vi "add_PointCloud_roslv.vi"(3 "channels":cluster{"name":string, "values":sgl[]}[](array[cluster]), 4 "points":cluster{"x":sgl, "y":sgl, "z":sgl}[](array[cluster]), 5 "frame_id":string, 6 "msg in":string) -> (2 "msg out":string)   [LabVIEW 2014]
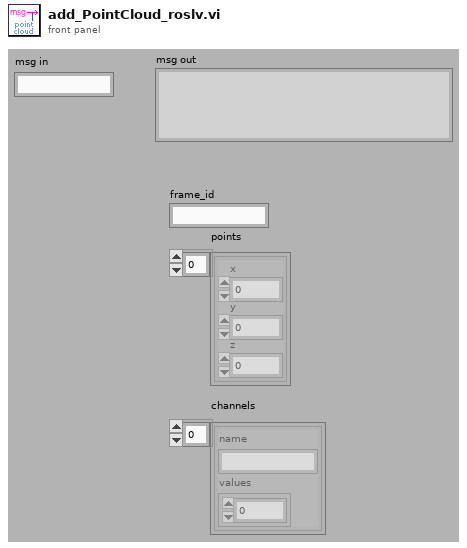
[diagram p1: front panel]
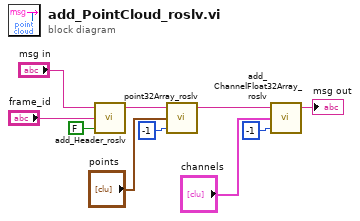
[diagram p0: block diagram]
diagram:
  n1 = call "add_Header_roslv.vi"("reset seq?"=FALSE, "frame_id"="frame_id", "msg in"="msg in") -> ("msg out"=w6:string)  [unwired: 2 in]
  n2 = call "point32Array_roslv.vi"("Array Length"=-1, "Array"="points", "msg in"=w6) -> ("msg out"=w2:string)  [unwired: 2 in]
  n3 = call "add_ChannelFloat32Array_roslv.vi"("Array Length"=-1, "Array"="channels", "msg in"=w2) -> ("msg out"=→"msg out":string)  [unwired: 2 in]
